vi "Configure Trigger.vi"(4 "External Trigger Slope (0: Positive)":u16(ring) items=["Positive", "Negative"], 6 "Internal Trigger Period (2 ms)":dbl[unit]=0.002, 8 "error in (no error)":errorcluster, 10 "Trigger Source (3:Internal)":u16(ring)=3 items=["Internal"=3, "External"=1], 11 "VISA resource name":refnum<visa-resource-name>) -> (0 "error out":errorcluster, 3 "VISA resource name out":refnum<visa-resource-name>)   [LabVIEW 2009, in "Tektronix AFG 3000 Series.lvlib"]
doc: "Configures the trigger source for triggering sweeps.\n\n<B>Note:</B> \n\nUse this VI only with other low-level VIs. The high-level VIs automatically incorporate this functionality."
uses:
  Tektronix AFG 3000 Series.lvlib
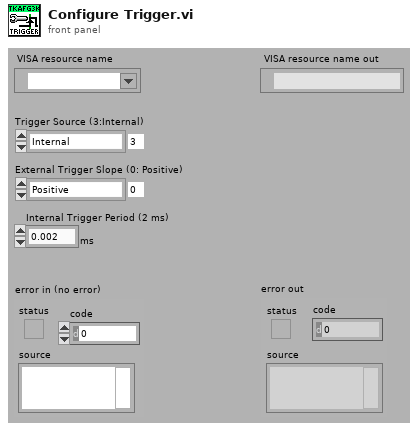
[diagram p1: front panel]
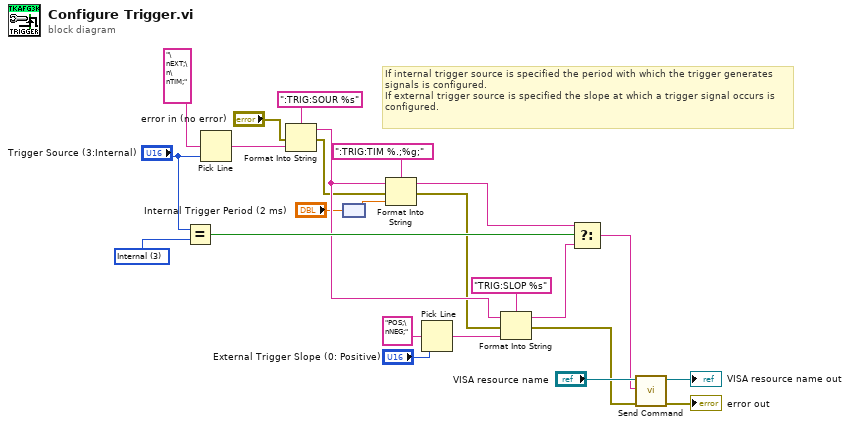
[diagram p0: block diagram]
diagram:
  w11 = u16 3 items=["Internal"=3, "External"=1] ("Trigger Source (3:Internal)")
  # "If internal trigger source is specified the period with which the trigger generates signals is configured.\nIf external trigger source is specified the slope at which a trigger signal occurs is configured."
  n1 = Equal?(x="Trigger Source (3:Internal)", y=w11) -> (x = y?=w20:bool)
  n2 = Pick Line(multi-line string="\nEXT;\n\nTIM;", line index="Trigger Source (3:Internal)") -> (output string=w23:string)  [unwired: 1 out]
  n3 = Format Into String(format string=":TRIG:SOUR %s", error in="error in (no error)", w23) -> (resulting string=w12:string, error out=w7:errorcluster)  [unwired: 1 in]
  n4 = node("Internal Trigger Period (2 ms)") -> (w9:dbl)
  n5 = Format Into String(format string=":TRIG:TIM %.;%g;", initial string=w12, error in=w7, w9) -> (resulting string=w21:string, error out=w6:errorcluster)
  n6 = Pick Line(multi-line string="POS;\nNEG;", line index="External Trigger Slope (0: Positive)") -> (output string=w18:string)  [unwired: 1 out]
  n7 = Format Into String(format string="TRIG:SLOP %s", initial string=w12, error in=w6, w18) -> (resulting string=w16:string, error out=w1:errorcluster)
  n8 = Select(t=w21, s=w20, f=w16) -> (s? t:f=w2:string)
  n9 = call "Send Command.vi"("error in (no error)"=w1, "write buffer"=w2, "VISA resource name"="VISA resource name") -> ("error out"=→"error out":errorcluster, "VISA resource name out"=→"VISA resource name out":refnum<visa-resource-name>)  [unwired: 7 out]
